vi "intensity_scaleHandler.vi"(9 "wavelengths":dbl[](array[numeric]), 10 "voltages":dbl[](array[numeric])) -> ()   [LabVIEW 2019]
uses:
  REFS.vi
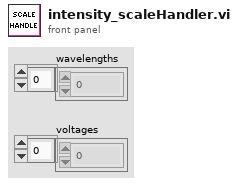
[diagram p1: front panel]
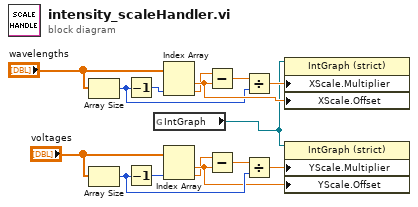
[diagram p0: block diagram]
diagram:
  n1 = Array Size(array="wavelengths") -> (size(s)=w12:i32)
  n2 = Array Size(array="voltages") -> (size(s)=w8:i32)
  n3 = Decrement(x=w12) -> (x-1=w10:i32)
  n4 = Decrement(x=w8) -> (x-1=w5:i32)
  n5 = global read "REFS.vi" "IntGraph"() -> (w1:refnum<vi>)
  n6 = Index Array(array="wavelengths", index #2=w10) -> (element #1=w14:dbl, element #2=w9:dbl)  [unwired: 1 in]
  n7 = Index Array(array="voltages", index #2=w5) -> (element #1=w4:dbl, element #2=w3:dbl)  [unwired: 1 in]
  n8 = Subtract(x=w9, y=w14) -> (x-y=w11:dbl)
  n9 = Subtract(x=w3, y=w4) -> (x-y=w7:dbl)
  n10 = Divide(x=w11, y=w12) -> (x/y=w13:dbl)
  n11 = Divide(x=w7, y=w8) -> (x/y=w6:dbl)
  n12 = property on="Property Node" class="IntGraph (strict)"(reference=w1, "XScale.Multiplier"=w13, "XScale.Offset"=w14) -> ()  [unwired: 1 in, 2 out]
  n13 = property on="Property Node" class="IntGraph (strict)"(reference=w1, "YScale.Multiplier"=w6, "YScale.Offset"=w4) -> ()  [unwired: 1 in, 2 out]
